vi "Open Method Front Panel.vi"(8 "error in (no error)":errorcluster, 10 "String":string, 11 "Execution UI In":refnum<class "Execution UI V2.lvclass">) -> (0 "error out":errorcluster, 3 "Execution UI Out":refnum<class "Execution UI V2.lvclass">)   [LabVIEW 2020]
uses:
  Execution UI V2.lvclass
  Execution UI V2.lvclass/Execution UI V2.ctl
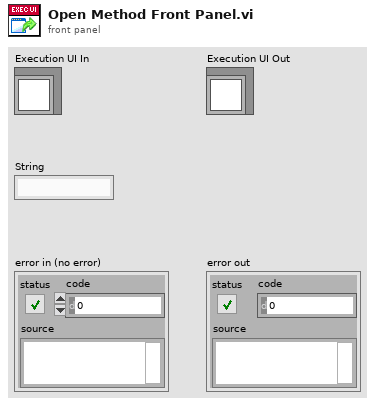
[diagram p1: front panel]
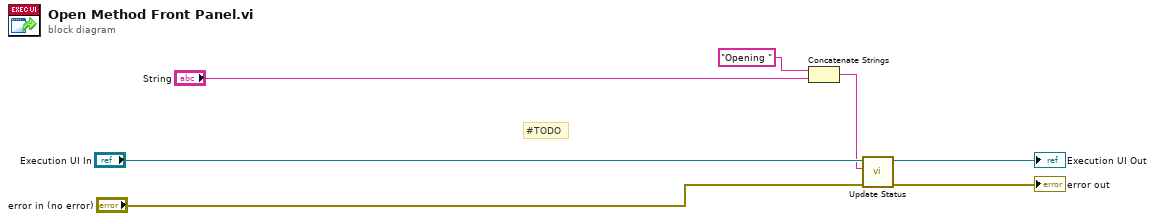
[diagram p0: block diagram]
diagram:
  # "#TODO"
  n1 = Concatenate Strings("Opening " ("string"), "String") -> (w1:string)
  n2 = call "Update Status.vi"("error in (no error)"="error in (no error)", "Status"=w1, "Execution UI In"="Execution UI In") -> ("error out"=→"error out":errorcluster, "Execution UI Out"=→"Execution UI Out":refnum<class "Execution UI V2.lvclass">)  [unwired: 7 in]
